vi "VI project.vi"() -> ()   [LabVIEW 2024]
uses:
  <vilib>/Analysis/3filter.llb/Filter Passband Type.ctl
  <vilib>/Analysis/baseanly.llb/Mean (DBL).vi
  <vilib>/Utility/file.llb/Read Delimited Spreadsheet (DBL).vi
  <vilib>/Analysis/3filter.llb/Butterworth Filter (DBL).vi
  <vilib>/Utility/file.llb/Write Delimited Spreadsheet (DBL).vi
  <vilib>/Analysis/NI_AALBase.lvlib
  <vilib>/Analysis/NI_AAL_SigProc.lvlib
panel:
  in  "stop":bool
  in  "Tab Control":T1(tab)
  out "Waveform Graph":dbl[](graph)
  out "Waveform Graph 2":dbl[](graph)
  out "Waveform Graph 3":dbl[](graph)
  out "Waveform Graph 4":dbl[](graph)
  out "Waveform Graph 5":dbl[](graph)
  out "Waveform Graph 6":dbl[](graph)
  out "Waveform Graph 7":dbl[](graph)
  out "Waveform Graph 8":dbl[](graph)
  out "Waveform Graph 9":dbl[][](graph)
  out "Waveform Graph 10":dbl[][](graph)
  out "Array":i32[](array[numeric])
  in  "Low Cutoff Freq":ext(slide)=5.0 scale=0.0..10.0
  in  "Sampling Frequency":dbl=1000.0 format="%0.2f"
  in  "file path (dialog if empty)":path
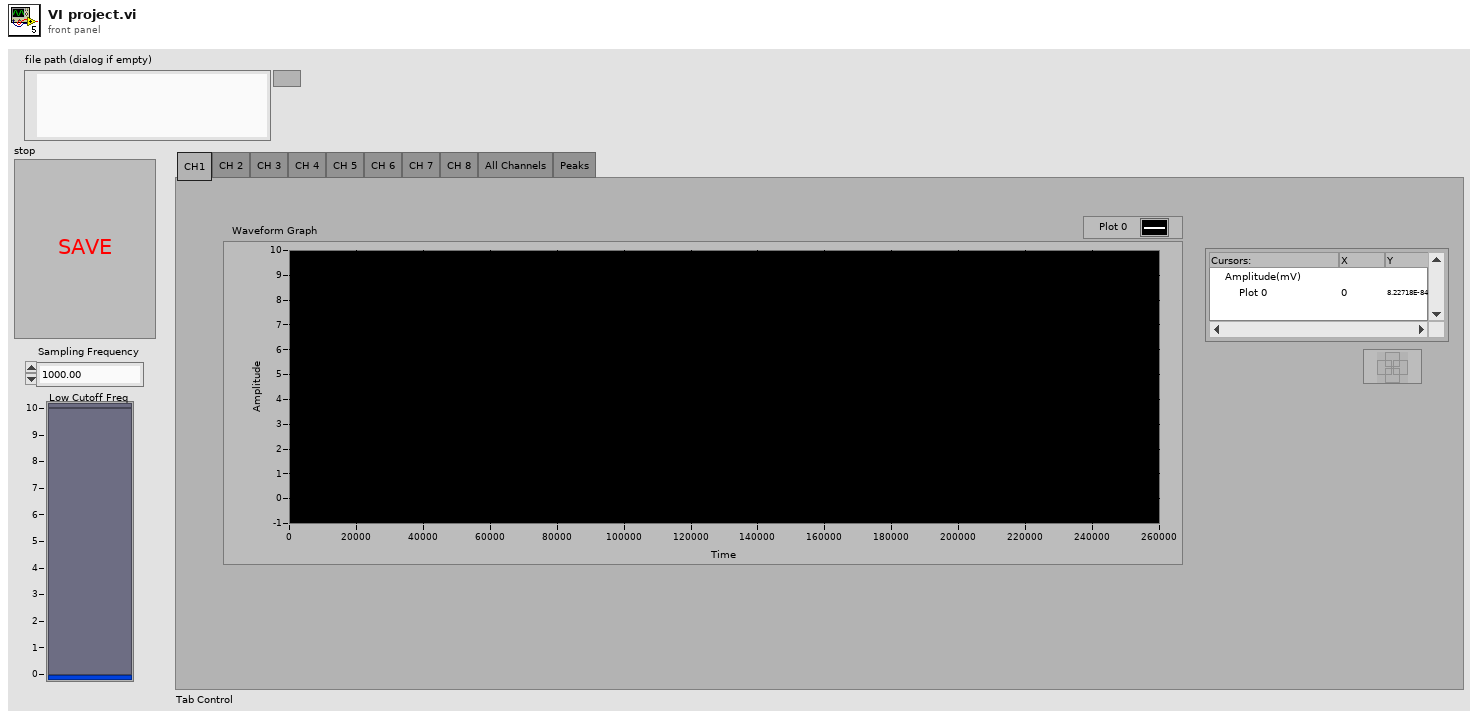
[diagram p1: front panel]
types:
  T1 = enum32{"CH1", "CH 2", "CH 3", "CH 4", "CH 5", "CH 6", "CH 7", "CH 8", "All Channels", "Peaks"}
  T2 = typedef "NI_AALBase.lvlib/Filter Passband Type.ctl" = enum32{"Lowpass", "Highpass", "Bandpass", "Bandstop"}
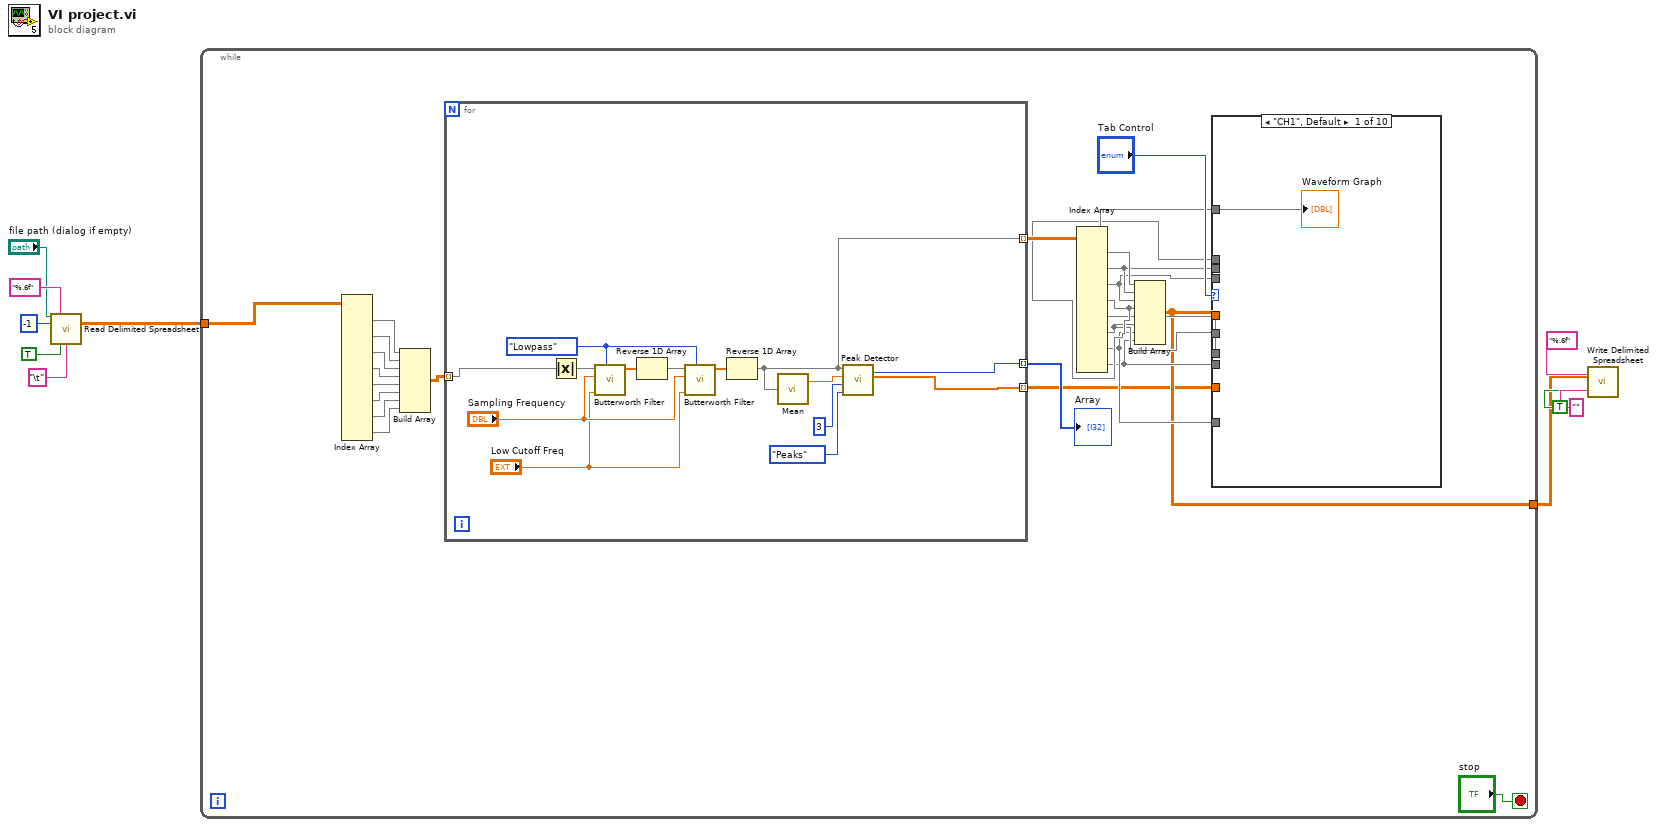
[diagram p0: block diagram]
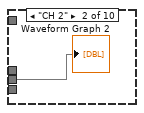
[diagram p2: hidden frame]
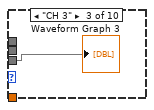
[diagram p3: hidden frame]
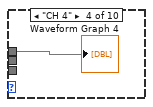
[diagram p4: hidden frame]
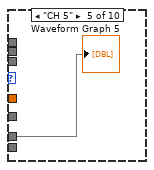
[diagram p5: hidden frame]
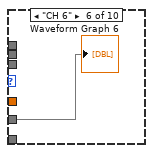
[diagram p6: hidden frame]
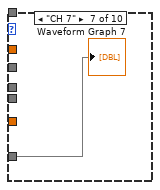
[diagram p7: hidden frame]
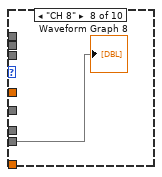
[diagram p8: hidden frame]
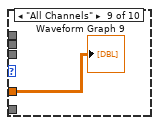
[diagram p9: hidden frame]
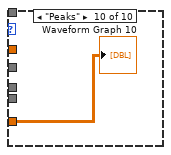
[diagram p10: hidden frame]
diagram:
  n1 = call-poly <vilib>:"Read Delimited Spreadsheet.vi"("file path (dialog if empty)"="file path (dialog if empty)", "format (%.3f)"="%.6f", "number of rows (all:-1)"=-1, "transpose? (F)"=TRUE, "delimiter (\\t)"="\t" ("delimiter (\\t)")) -> ("all rows"=w5:dbl[][])  [unwired: 5 in, 5 out]
  n2 = while {
    tunnel: w5 -> [w34]
    tunnel: [w13] -> w1
    stop <- "stop" stop-if-true
    n3 = Index Array(array=w34) -> (element #1=w33:dbl[], element #2=w32:dbl[], element #3=w31:dbl[], element #4=w30:dbl[], element #5=w29:dbl[], element #6=w28:dbl[], element #7=w27:dbl[], element #8=w26:dbl[])  [unwired: 16 in]
    n4 = Build Array(w33, w32, w31, w30, w29, w28, w27, w26) -> (w25:dbl[][])
    n5 = for {
      tunnel: w25 -> [w58] mode=indexing
      tunnel: [w47] -> w24 mode=indexing
      tunnel: [w46] -> w23 mode=indexing
      tunnel: [w45] -> w12 mode=indexing
      w53 = Filter_Passband_Type."Lowpass" ("filter type")
      n6 = Absolute Value(x=w58) -> (abs(x)=w57:dbl[])
      n7 = call-poly <vilib>:"Butterworth Filter.vi"("filter type"=w53, "low cutoff freq: fl"="Low Cutoff Freq", "sampling freq: fs"="Sampling Frequency", "X"=w57) -> ("Filtered X"=w56:dbl[])  [unwired: 4 in, 1 out]
      n8 = Reverse 1D Array(array=w56) -> (reversed array=w54:dbl[])
      n9 = call-poly <vilib>:"Butterworth Filter.vi"("filter type"=w53, "low cutoff freq: fl"="Low Cutoff Freq", "sampling freq: fs"="Sampling Frequency", "X"=w54) -> ("Filtered X"=w55:dbl[])  [unwired: 4 in, 1 out]
      n10 = Reverse 1D Array(array=w55) -> (reversed array=w47:dbl[])
      n11 = call-poly <vilib>:"Mean.vi"("X"=w47) -> ("mean"=w50:dbl)  [unwired: 1 out]
      n12 = call <vilib>:"Peak Detector.vi"("peaks/valleys"=enum32{"Peaks", "Valleys"}."Peaks", "width"=3, "threshold"=w50, "X"=w47) -> ("Amplitudes"=w45:dbl[], "# found"=w46:i32)  [unwired: 3 in, 3 out]
    }
    "Array" <- w23
    n13 = Index Array(array=w24) -> (element #1=w21:dbl[], element #2=w20:dbl[], element #3=w19:dbl[], element #4=w18:dbl[], element #5=w17:dbl[], element #6=w16:dbl[], element #7=w15:dbl[], element #8=w14:dbl[])  [unwired: 16 in]
    n14 = Build Array(w21, w20, w19, w18, w17, w16, w15, w14) -> (w13:dbl[][])
    n15 = case shown="\"CH1\", Default" "Tab Control" {
      tunnel: w21 -> [w35 _ _ _ _ _ _ _ _ _]
      tunnel: w20 -> [_ w36 _ _ _ _ _ _ _ _]
      tunnel: w19 -> [_ _ w37 _ _ _ _ _ _ _]
      tunnel: w18 -> [_ _ _ w38 _ _ _ _ _ _]
      tunnel: w17 -> [_ _ _ _ w39 _ _ _ _ _]
      tunnel: w16 -> [_ _ _ _ _ w40 _ _ _ _]
      tunnel: w15 -> [_ _ _ _ _ _ w41 _ _ _]
      tunnel: w14 -> [_ _ _ _ _ _ _ w42 _ _]
      tunnel: w13 -> [_ _ _ _ _ _ _ _ w43 _]
      tunnel: w12 -> [_ _ _ _ _ _ _ _ _ w44]
      frame "CH1", Default {
        "Waveform Graph" <- w35
      }
      frame "CH 2" {
        "Waveform Graph 2" <- w36
      }
      frame "CH 3" {
        "Waveform Graph 3" <- w37
      }
      frame "CH 4" {
        "Waveform Graph 4" <- w38
      }
      frame "CH 5" {
        "Waveform Graph 5" <- w39
      }
      frame "CH 6" {
        "Waveform Graph 6" <- w40
      }
      frame "CH 7" {
        "Waveform Graph 7" <- w41
      }
      frame "CH 8" {
        "Waveform Graph 8" <- w42
      }
      frame "All Channels" {
        "Waveform Graph 9" <- w43
      }
      frame "Peaks" {
        "Waveform Graph 10" <- w44
      }
    }
  }
  n16 = call-poly <vilib>:"Write Delimited Spreadsheet.vi"("format (%.3f)"="%.6f", "2D data"=w1, "transpose? (no:F)"=TRUE, "delimiter (\\t)"="" ("delimiter (\\t)")) -> ()  [unwired: 10 in, 2 out]
